vi "MultiplyTwoNumbers.vi"() -> ()   [LabVIEW 2015]
panel:
  out "Product":dbl
  in  "Number 2":dbl
  in  "Number 1":dbl
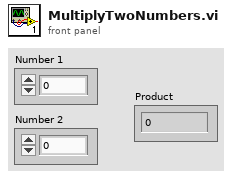
[diagram p1: front panel]
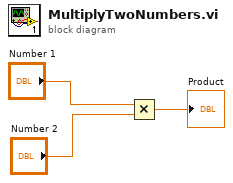
[diagram p0: block diagram]
diagram:
  n1 = Multiply(x="Number 1", y="Number 2") -> (x*y=→"Product":dbl)
